vi "Front Panel to System Tray.vi"(6 "Balloon Tip Information":T1, 7 "Mode":enum16{"Enabled", "Disabled"}(ring), 8 "error in":errorcluster, 10 "VIRef":refnum<vi>, 11 "NotifyIcon":refnum<class "NotifyIcon.lvclass">) -> (0 "error out":errorcluster, 3 "NotifyIcon":refnum<class "NotifyIcon.lvclass">)   [LabVIEW 2014]
doc: "<B>Copyright</B>: (c) 2015 MHWirth. All rights reserved.\n\nThis subVI hides the front panel and makes the icon visible in system tray. This cab be called in \"Panel Resized\" event when action is \"minimized\".\n\nTo remove the page from the taskbar in <B>executable</B> the following two properties must be in the config file in the section with the same name as the executable name.\n\nHideRootWindow = TRUE\nallowmultipleinstances = TRUE"
uses:
  <userlib>/Notify Icon/Public/NotifyIcon.lvclass
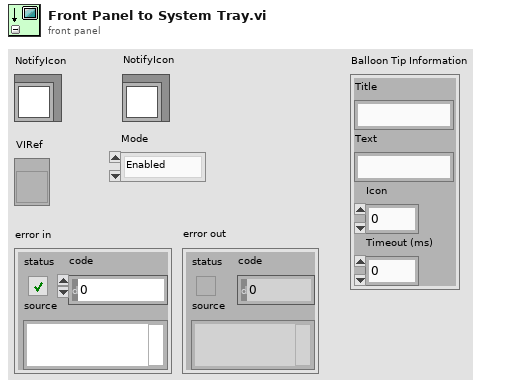
[diagram p1: front panel]
types:
  T1 = cluster{"Title":string, "Text":string, "Icon":i32, "Timeout (ms)":i32}
  T2 = enum32{"Invalid", "Standard", "Closed", "Hidden", "Minimized", "Maximized"}
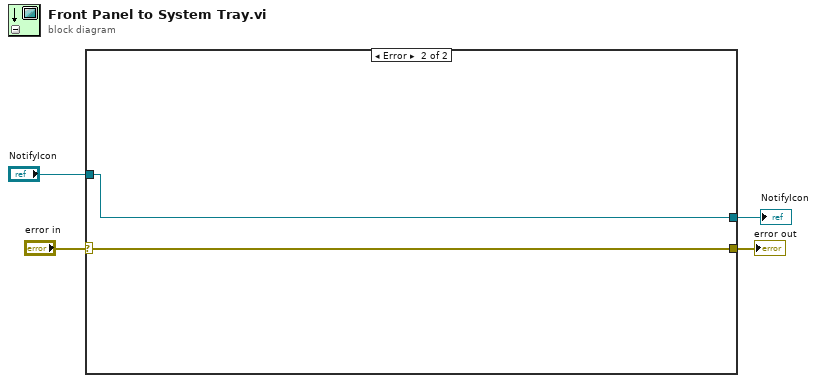
[diagram p0: block diagram]
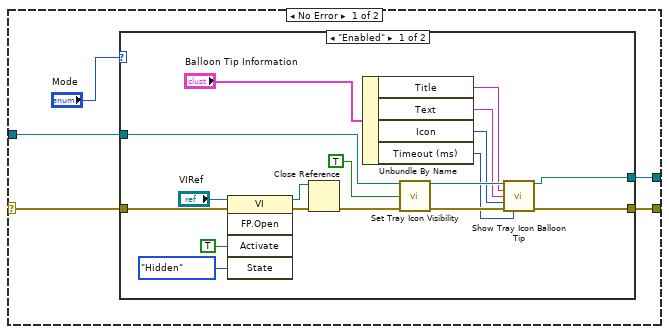
[diagram p2: hidden frame]
diagram:
  n1 = case shown="Error" "error in" {
    selector: "error in" -> [w9 w31]
    tunnel: [w8 w31] -> w3
    tunnel: "NotifyIcon" -> [w6 w30]
    tunnel: [w5 w30] -> w1
    frame No Error {
      n2 = case shown="\"Enabled\"" "Mode" {
        tunnel: w9 -> [w18 w29]
        tunnel: [w12 w29] -> w8
        tunnel: w6 -> [w11 w28]
        tunnel: [w10 w28] -> w5
        frame "Enabled" {
          n3 = invoke class="VI" method="FP.Open"(reference="VIRef", error in=w18, "Activate"=TRUE ("Activate?"), "State"=T2."Hidden") -> (reference out=w25:refnum<vi>, error out=w26:errorcluster)  [unwired: 1 in, 3 out]
          n4 = Close Reference(reference=w25, error in (no error)=w26) -> (error out=w24:errorcluster)
          n5 = Unbundle By Name("Balloon Tip Information") -> ("Title"=w16:string, "Text"=w15:string, "Icon"=w14:i32, "Timeout (ms)"=w13:i32)
          n6 = call <userlib>:"Set Tray Icon Visibility.vi"("NotifyIcon in"=w11, "Show Tray Icon"=TRUE, "error in (no error)"=w24) -> ("NotifyIcon out"=w21:refnum<class "NotifyIcon.lvclass">, "error out"=w22:errorcluster)  [unwired: 11 out]
          n7 = call <userlib>:"Show Tray Icon Balloon Tip.vi"("NotifyIcon in"=w21, "Title"=w16, "Text"=w15, "Icon"=w14, "error in (no error)"=w22, "Timeout (ms)"=w13) -> ("NotifyIcon out"=w10:refnum<class "NotifyIcon.lvclass">, "error out"=w12:errorcluster)  [unwired: 8 out]
        }
        frame "Disabled", Default {
        }
      }
    }
    frame Error {
    }
  }
  "error out" <- w3
  "NotifyIcon" <- w1
